vi "isReporting.vi"(8 "error in (no error)":errorcluster, 11 "Test Report.Template in":refnum<class "Test Report.Template.lvclass">) -> (0 "error out":errorcluster, 2 "Exporting?":bool, 3 "Test Report.Template out":refnum<class "Test Report.Template.lvclass">)   [LabVIEW 2013, in "Caraya.lvlib" / "Test Report.Template.lvclass"]
uses:
  Test Report.Template.lvclass
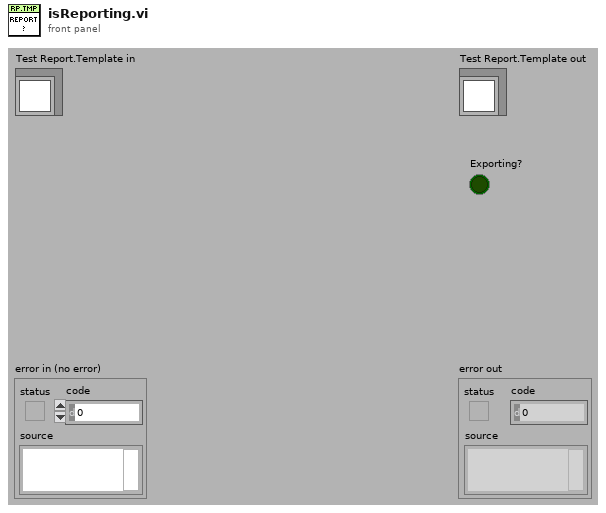
[diagram p1: front panel]
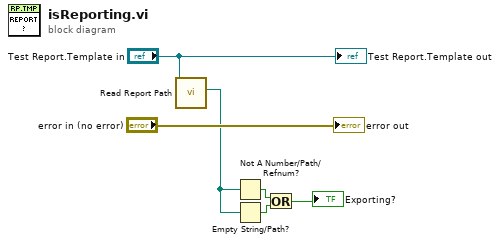
[diagram p0: block diagram]
diagram:
  n1 = call "Read Report Path.vi"("Test Report.Default in"="Test Report.Template in") -> ("Report Path"=w2:path)  [unwired: 9 in, 1 out]
  n2 = Not A Number/Path/Refnum?(number/path/refnum=w2) -> (NaN/Path/Refnum?=w5:bool)
  n3 = Empty String/Path?(string/path=w2) -> (empty?=w6:bool)
  n4 = Or(x=w5, y=w6) -> (x .or. y?=→"Exporting?":bool)
  "error out" <- "error in (no error)"
  "Test Report.Template out" <- "Test Report.Template in"
